vi "General Config.vi"(8 "error In":errorcluster, 9 "DO":T1, 10 "IOList":T3, 11 "reference":refnum<vi>) -> (0 "error out":errorcluster, 3 "Out reference":refnum<vi>)   [LabVIEW 2015]
uses:
  Control Button/Exit.ctl
  Control Button/Daq.ctl
  Control Button/Scanner config.ctl
  Control Button/Program Seq.ctl
  Control Button/Control 1.ctl
  Control Button/cali.ctl
  Control Button/shift change.ctl
  Control Button/User mgt.ctl
  Control Button/model create.ctl
  Data Acquisition/PCI-USB-DAQ/Digital out put.ctl
  Galobal variable_TI.vi
panel:
  out "User Name 3":string
  in  "Model Create":T2
  in  "User Mgt":T4
  out "User Name 2":string
  in  "Shift":T5
  in  "Calibration":T6
  in  "IO List Update":T7
  out "error out 2":errorcluster
  in  "error in (no error)":errorcluster
  in  "Program Seq":T8
  in  "Scanner config":T9
  in  "DAQ Config":T10
  out "User Name":string
  in  "Exit":T11
  out "String":string
  out "appended path":path
  in  "Ring":u16(ring)
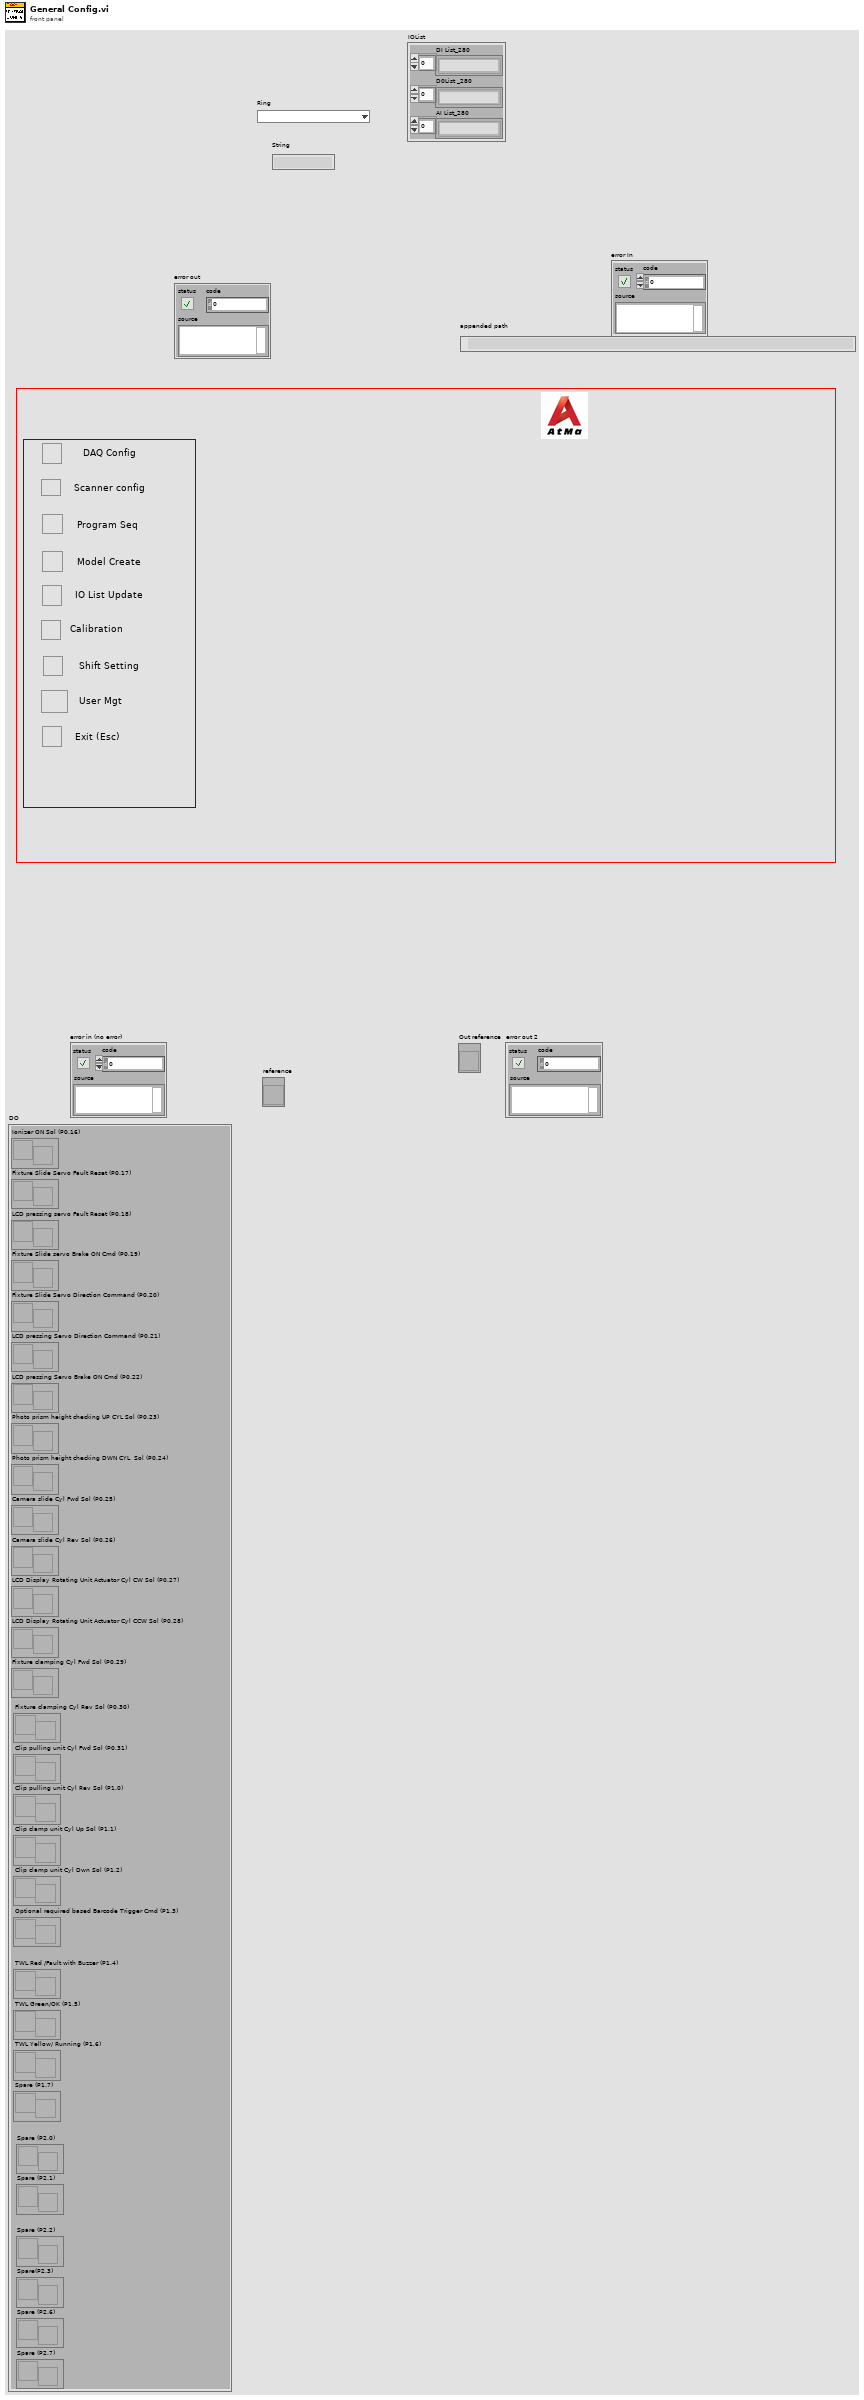
[diagram p1: front panel]
types:
  T1 = typedef "Digital out put.ctl" = cluster{"Ionizer ON Sol (P0.16)":refnum<notifier>, "Fixture Slide Servo Fault Reset (P0.17)":refnum<notifier>, "LCD pressing servo Fault Reset (P0.18)":refnum<notifier>, "Fixture Slide servo Brake ON Cmd (P0.19)":refnum<notifier>, "Fixture Slide Servo Direction Command (P0.20)":refnum<notifier>, "LCD pressing Servo Direction Command (P0.21)":refnum<notifier>, "LCD pressing Servo Brake ON Cmd (P0.22)":refnum<notifier>, "Photo prism height checking UP CYL Sol (P0.23)":refnum<notifier>, "Photo prism height checking DWN CYL  Sol (P0.24)":refnum<notifier>, "Camera slide Cyl Fwd Sol (P0.25)":refnum<notifier>, "Camera slide Cyl Rev Sol (P0.26)":refnum<notifier>, "LCD Display Rotating Unit Actuator Cyl CW Sol (P0.27)":refnum<notifier>, "LCD Display Rotating Unit Actuator Cyl CCW Sol (P0.28)":refnum<notifier>, "Fixture clamping Cyl Fwd Sol (P0.29)":refnum<notifier>, "Fixture clamping Cyl Rev Sol (P0.30)":refnum<notifier>, "Clip pulling unit Cyl Fwd Sol (P0.31)":refnum<notifier>, "Clip pulling unit Cyl Rev Sol (P1.0)":refnum<notifier>, "Clip clamp unit Cyl Up Sol (P1.1)":refnum<notifier>, "Clip clamp unit Cyl Dwn Sol (P1.2)":refnum<notifier>, "Optional required based Barcode Trigger Cmd (P1.3)":refnum<notifier>, "TWL Red /Fault with Buzzer (P1.4)":refnum<notifier>, "TWL Green/OK (P1.5)":refnum<notifier>, "TWL Yellow/ Running (P1.6)":refnum<notifier>, "Spare (P1.7)":refnum<notifier>, "Spare (P2.0)":refnum<notifier>, "Spare (P2.1)":refnum<notifier>, "Spare (P2.2)":refnum<notifier>, "Spare(P2.3)":refnum<notifier>, "Spare (P2.6)":refnum<notifier>, "Spare (P2.7) ":refnum<notifier>}
  T2 = typedef "model create.ctl" = bool
  T3 = cluster{"DI List_280":string[], "D0List _280":string[], "AI List_280":string[]}
  T4 = typedef "User mgt.ctl" = bool
  T5 = typedef "shift change.ctl" = bool
  T6 = typedef "cali.ctl" = bool
  T7 = typedef "Control 1.ctl" = bool
  T8 = typedef "Program Seq.ctl" = bool
  T9 = typedef "Scanner config.ctl" = bool
  T10 = typedef "Daq.ctl" = bool
  T11 = typedef "Exit.ctl" = bool
  T12 = enum32{"Invalid", "Standard", "Closed", "Hidden", "Minimized", "Maximized"}
  T13 = cluster{"XInput":dbl[], "Y New Value":dbl[], "Avg point":i16}[]
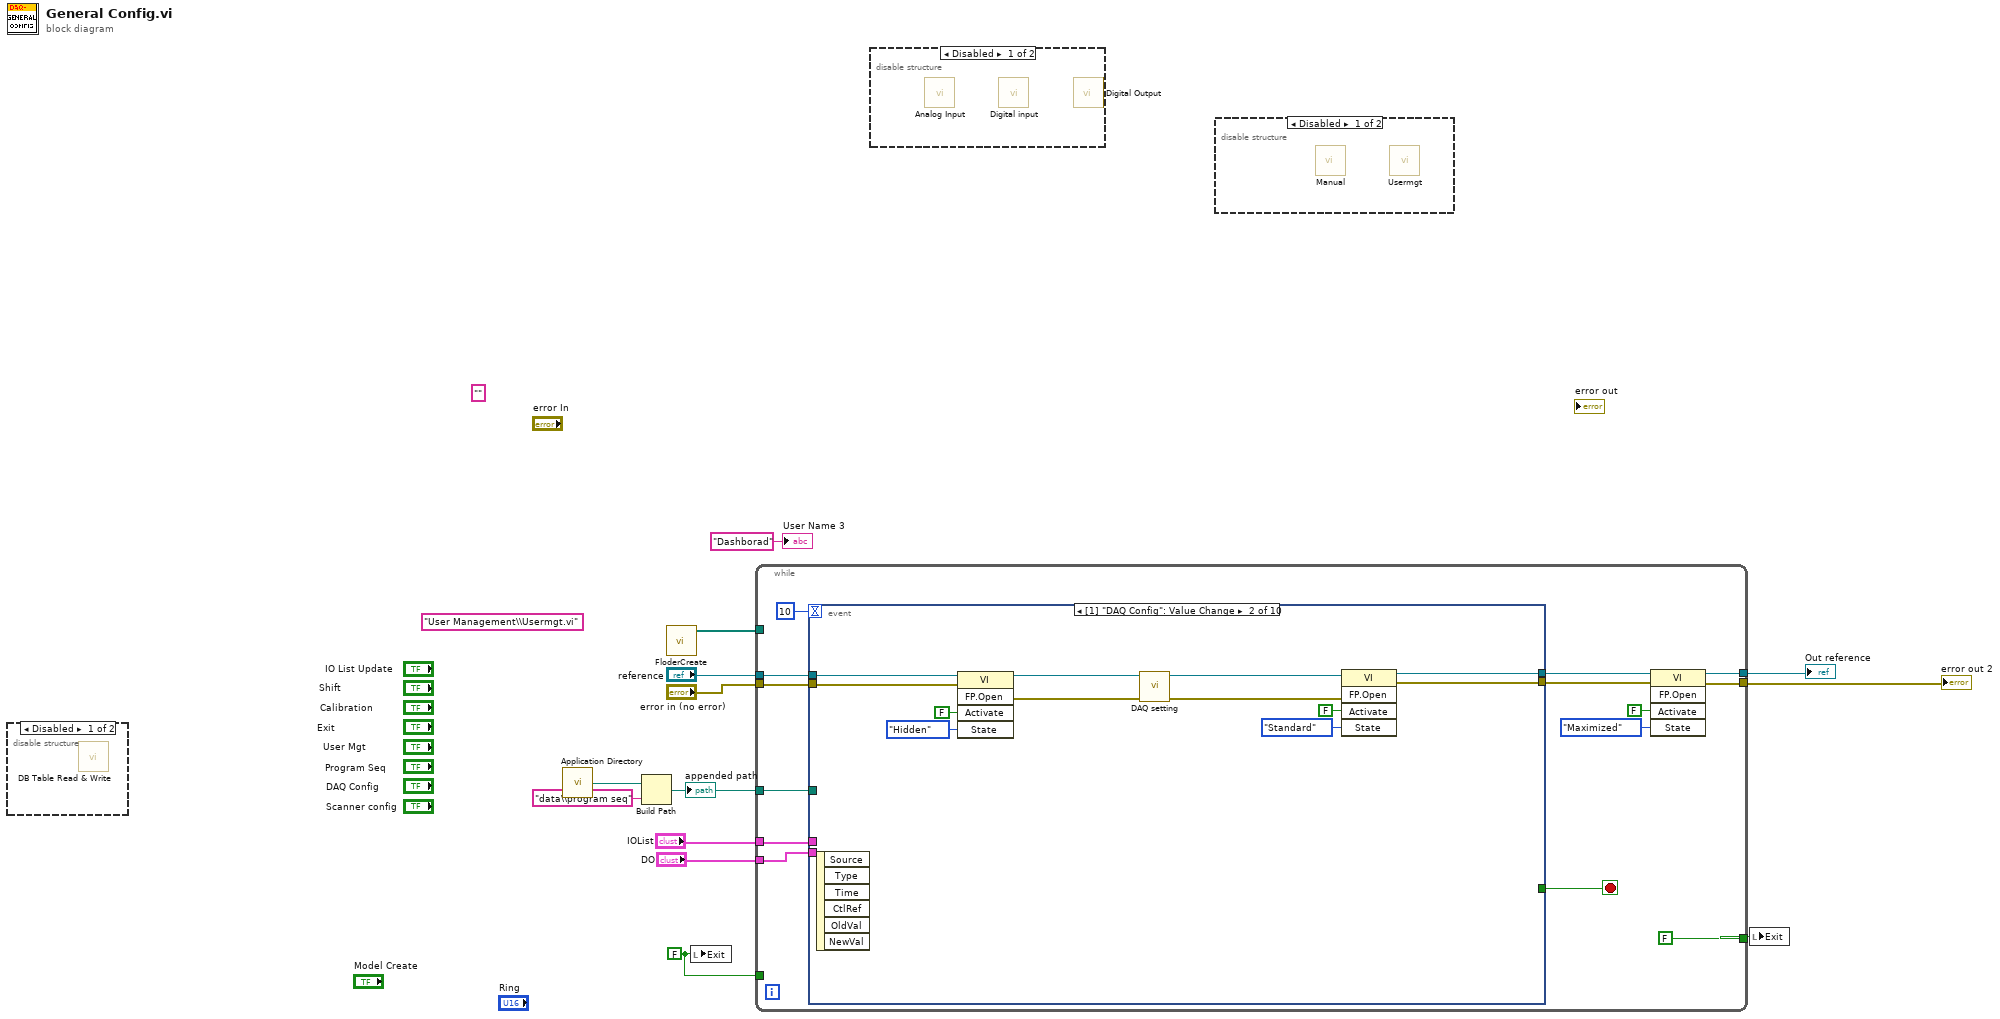
[diagram p0: block diagram]
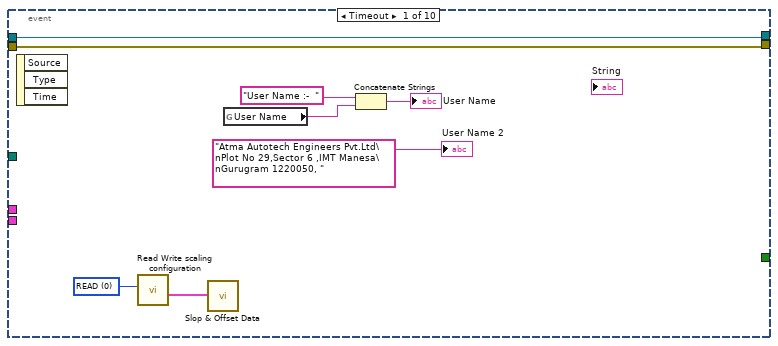
[diagram p5: hidden frame]
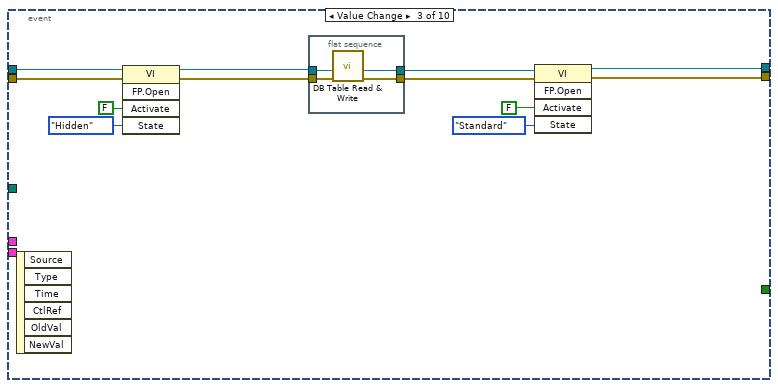
[diagram p6: hidden frame]
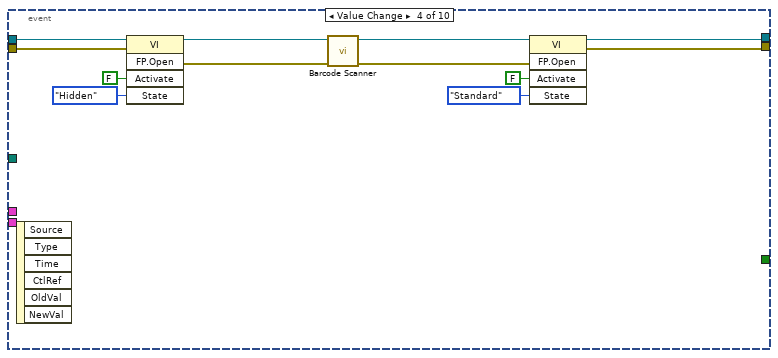
[diagram p7: hidden frame]
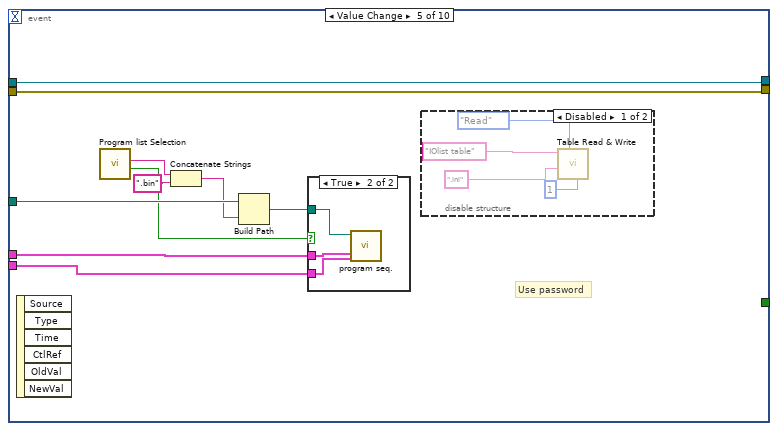
[diagram p8: hidden frame]
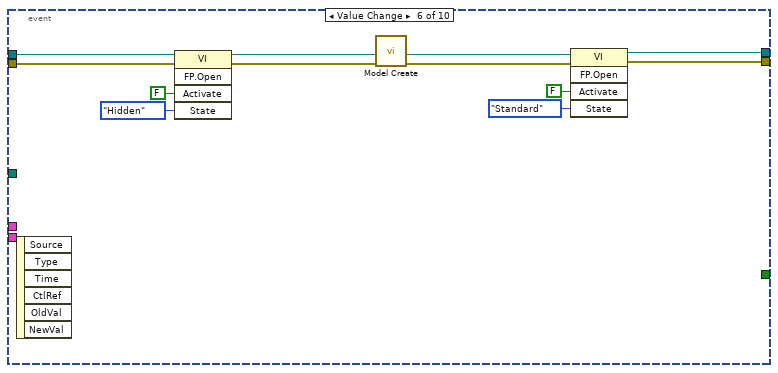
[diagram p11: hidden frame]
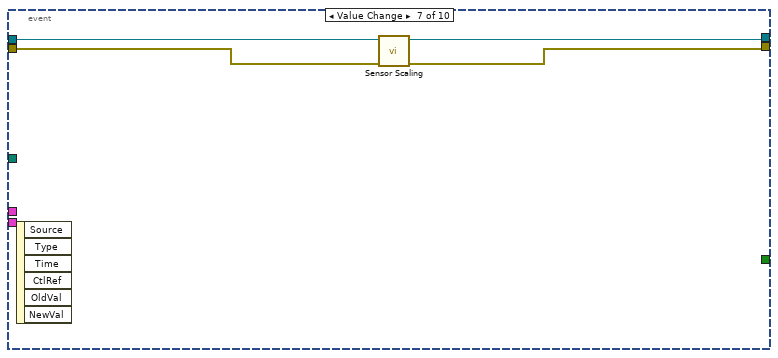
[diagram p12: hidden frame]
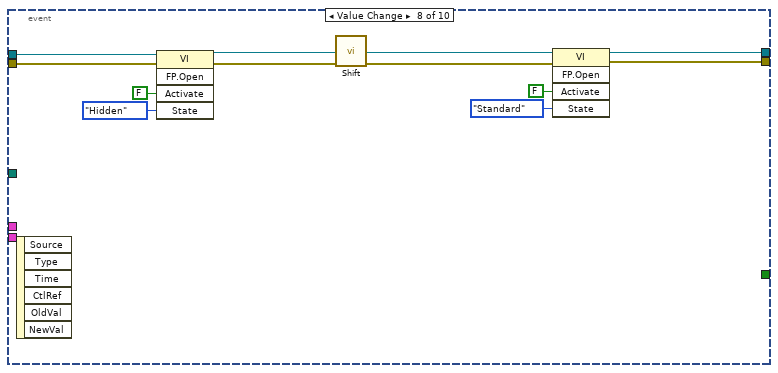
[diagram p13: hidden frame]
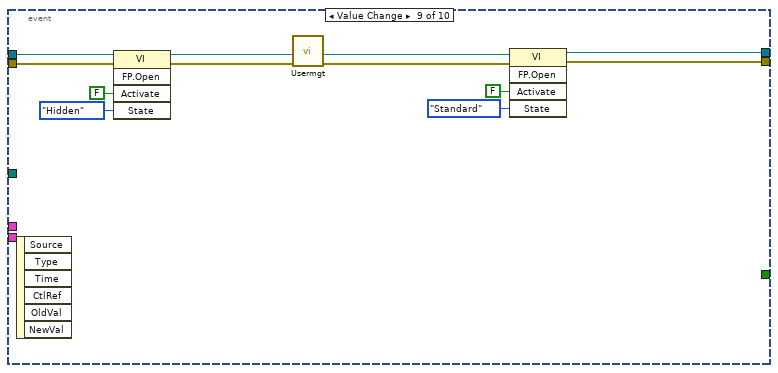
[diagram p14: hidden frame]
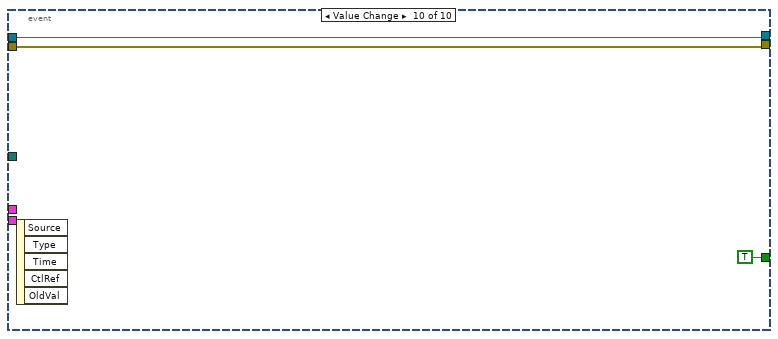
[diagram p15: hidden frame]
diagram:
  w10 = T11 FALSE ("Exit")
  (unwired) "User Management\\Usermgt.vi" ("name or relative path")
  (unwired) ""
  n1 = disable-structure shown="Disabled" {
    frame Disabled {
      n2 = call "DB Table Read & Write.vi"() -> ()  [unwired: 10 in, 2 out]
    }
    frame Enabled {
    }
  }
  n3 = call <vilib>:"Application Directory.vi"() -> ("Application Directory"=w6:path)
  n4 = Build Path(base path=w6, name or relative path="data\\program seq") -> (appended path=w3:path)
  "appended path" <- w3
  n5 = call "FloderCreate.vi"() -> ("File Path"=w7:path[])  [unwired: 11 in]
  n6 = local write "Exit"(w10) -> ()
  n7 = while {
    tunnel: w3 -> [w15]
    tunnel: "reference" -> [w25]
    tunnel: "error in (no error)" -> [w24]
    tunnel: [w19] -> w12
    tunnel: [w18] -> w11
    tunnel: w10 -> [_]
    tunnel: [T11 FALSE ("Exit")] -> w9
    tunnel: w7 -> [_]
    tunnel: "IOList" -> [w16]
    tunnel: "DO" -> [w14]
    stop <- w26 stop-if-true
    n8 = event shown="[1] \"DAQ Config\": Value Change" {
      selector: _ -> [_ _ _ _ _ _ _ _ _ _]
      dyn-events: _ -> [_ _ _ _ _ _ _ _ _ _]
      timeout: 10 -> [_ _ _ _ _ _ _ _ _ _]
      tunnel: [_ _ _ _ _ _ _ _ _ TRUE ("Exit")] -> w26
      tunnel: w25 -> [w32 w39 w51 w73 w85 w99 w106 w114 w123 w131]
      tunnel: w24 -> [w31 w38 w50 w72 w84 w98 w105 w112 w121 w130]
      tunnel: [w32 w37 w58 w65 w85 w94 w106 w113 w122 w131] -> w21
      tunnel: [w31 w36 w57 w64 w84 w93 w104 w111 w120 w130] -> w20
      tunnel: w16 -> [_ _ _ _ w83 _ _ _ _ _]
      tunnel: w15 -> [_ _ _ _ w82 _ _ _ _ _]
      tunnel: w14 -> [_ _ _ _ w76 _ _ _ _ _]
      event Timeout {
        w30 = u16 0 items=["READ", "WRITE"] ("Read/Write")
        n9 = event-data() -> ()  [unwired: 1 in, 3 out]
        n10 = call "Read Write scaling configuration.vi"("Read/Write"=w30) -> ("Output"=w29:T13)  [unwired: 4 in, 2 out]
        n11 = call "Slop & Offset Data.vi"("Input"=w29) -> ()  [unwired: 10 in, 1 out]
        n12 = global read "Galobal variable_TI.vi" "User Name"() -> (w35:string)
        n13 = Concatenate Strings("User Name :-  " ("string"), w35) -> (→"User Name":string)
        "User Name 2" <- "Atma Autotech Engineers Pvt.Ltd\nPlot No 29,Sector 6 ,IMT Manesa\nGurugram 1220050, " ("string")
      }
      event Value Change {
        n14 = event-data() -> ()  [unwired: 1 in, 6 out]
        n15 = invoke class="VI" method="FP.Open"(reference=w39, error in=w38, "Activate"=FALSE ("Activate?"), "State"=T12."Hidden") -> (reference out=w45:refnum<vi>, error out=w44:errorcluster)  [unwired: 1 in, 3 out]
        n16 = call "DAQ setting.vi"("error in (no error)"=w44, "vi reference"=w45) -> ("error Out"=w40:errorcluster, "Out reference"=w41:refnum<vi>)  [unwired: 8 in]
        n17 = invoke class="VI" method="FP.Open"(reference=w41, error in=w40, "Activate"=FALSE ("Activate?"), "State"=T12."Standard") -> (reference out=w37:refnum<vi>, error out=w36:errorcluster)  [unwired: 1 in, 3 out]
      }
      event Value Change {
        n18 = event-data() -> ()  [unwired: 1 in, 6 out]
        n19 = invoke class="VI" method="FP.Open"(reference=w51, error in=w50, "Activate"=FALSE ("Activate?"), "State"=T12."Hidden") -> (reference out=w49:refnum<vi>, error out=w48:errorcluster)  [unwired: 1 in, 3 out]
        n20 = flat-sequence {
          tunnel: [w60] -> w55
          tunnel: [w61] -> w54
          tunnel: w49 -> [w62]
          tunnel: w48 -> [w63]
          frame #0 {
            n21 = call "DB Table Read & Write.vi"("error in"=w63, "reference"=w62) -> ("error out"=w60:errorcluster, "referenceOut"=w61:refnum<vi>)  [unwired: 8 in]
          }
        }
        n22 = invoke class="VI" method="FP.Open"(reference=w54, error in=w55, "Activate"=FALSE ("Activate?"), "State"=T12."Standard") -> (reference out=w58:refnum<vi>, error out=w57:errorcluster)  [unwired: 1 in, 3 out]
      }
      event Value Change {
        n23 = event-data() -> ()  [unwired: 1 in, 6 out]
        n24 = invoke class="VI" method="FP.Open"(reference=w73, error in=w72, "Activate"=FALSE ("Activate?"), "State"=T12."Hidden") -> (reference out=w69:refnum<vi>, error out=w68:errorcluster)  [unwired: 1 in, 3 out]
        n25 = call "Barcode Scanner.vi"("error in (no error)"=w68, "reference"=w69) -> ("error in (no error) 2"=w66:errorcluster, "reference 2"=w67:refnum<vi>)  [unwired: 8 in]
        n26 = invoke class="VI" method="FP.Open"(reference=w67, error in=w66, "Activate"=FALSE ("Activate?"), "State"=T12."Standard") -> (reference out=w65:refnum<vi>, error out=w64:errorcluster)  [unwired: 1 in, 3 out]
      }
      event Value Change {
        # "Use password"
        n27 = event-data() -> ()  [unwired: 1 in, 6 out]
        n28 = call "Program list Selection.vi"() -> ("Exit"=w77:bool, "String"=w78:string)  [unwired: 10 in]
        n29 = Concatenate Strings(w78, ".bin" ("string")) -> (w81:string)
        n30 = Build Path(base path=w82, name or relative path=w81) -> (appended path=w79:path)
        n31 = case shown="True" w77 {
          tunnel: w83 -> [_ w86]
          tunnel: w79 -> [_ w88]
          tunnel: w76 -> [_ w87]
          frame False {
          }
          frame True {
            n32 = call "program seq..vi"("IOList"=w86, "DO"=w87, "Filepath"=w88) -> ()  [unwired: 8 in, 1 out]
          }
        }
        n33 = disable-structure shown="Disabled" {
          frame Disabled {
            n34 = call "Table Read & Write.vi"("File Name"="IOlist table", "File type"=".ini", "Enum"=enum16{"Read", "Write"}."Read", "index"=1) -> ()  [unwired: 5 in, 2 out]
          }
          frame Enabled {
          }
        }
      }
      event Value Change {
        n35 = event-data() -> ()  [unwired: 1 in, 6 out]
        n36 = invoke class="VI" method="FP.Open"(reference=w99, error in=w98, "Activate"=FALSE ("Activate?"), "State"=T12."Hidden") -> (reference out=w95:refnum<vi>, error out=w97:errorcluster)  [unwired: 1 in, 3 out]
        n37 = call "Model Create.vi"("error in (no error)"=w97) -> ("error out"=w96:errorcluster)  [unwired: 10 in]
        n38 = invoke class="VI" method="FP.Open"(reference=w95, error in=w96, "Activate"=FALSE ("Activate?"), "State"=T12."Standard") -> (reference out=w94:refnum<vi>, error out=w93:errorcluster)  [unwired: 1 in, 3 out]
      }
      event Value Change {
        n39 = event-data() -> ()  [unwired: 1 in, 6 out]
        n40 = call "Sensor Scaling.vi"("error in"=w105) -> ("error out"=w104:errorcluster)  [unwired: 9 in, 1 out]
      }
      event Value Change {
        n41 = event-data() -> ()  [unwired: 1 in, 6 out]
        n42 = invoke class="VI" method="FP.Open"(reference=w114, error in=w112, "Activate"=FALSE ("Activate?"), "State"=T12."Hidden") -> (reference out=w115:refnum<vi>, error out=w117:errorcluster)  [unwired: 1 in, 3 out]
        n43 = call "Shift.vi"("error in"=w117) -> ("error out"=w116:errorcluster)  [unwired: 10 in]
        n44 = invoke class="VI" method="FP.Open"(reference=w115, error in=w116, "Activate"=FALSE ("Activate?"), "State"=T12."Standard") -> (reference out=w113:refnum<vi>, error out=w111:errorcluster)  [unwired: 1 in, 3 out]
      }
      event Value Change {
        n45 = event-data() -> ()  [unwired: 1 in, 6 out]
        n46 = invoke class="VI" method="FP.Open"(reference=w123, error in=w121, "Activate"=FALSE ("Activate?"), "State"=T12."Hidden") -> (reference out=w124:refnum<vi>, error out=w119:errorcluster)  [unwired: 1 in, 3 out]
        n47 = call "Usermgt.vi"("error In"=w119) -> ("error out"=w118:errorcluster)  [unwired: 10 in]
        n48 = invoke class="VI" method="FP.Open"(reference=w124, error in=w118, "Activate"=FALSE ("Activate?"), "State"=T12."Standard") -> (reference out=w122:refnum<vi>, error out=w120:errorcluster)  [unwired: 1 in, 3 out]
      }
      event Value Change {
        n49 = event-data() -> ()  [unwired: 1 in, 5 out]
      }
    }
    n50 = invoke class="VI" method="FP.Open"(reference=w21, error in=w20, "Activate"=FALSE ("Activate?"), "State"=T12."Maximized") -> (reference out=w19:refnum<vi>, error out=w18:errorcluster)  [unwired: 1 in, 3 out]
  }
  "Out reference" <- w12
  "error out 2" <- w11
  n51 = disable-structure shown="Disabled" {
    frame Disabled {
      n52 = call "Analog Input.vi"() -> ()  [unwired: 10 in, 2 out]
      n53 = call "Digital input.vi"() -> ()  [unwired: 10 in, 2 out]
      n54 = call "Digital Output.vi"() -> ()  [unwired: 10 in, 2 out]
    }
    frame Enabled {
    }
  }
  n55 = disable-structure shown="Disabled" {
    frame Disabled {
      n56 = call "Manual.vi"() -> ()  [unwired: 10 in, 2 out]
      n57 = call "Usermgt.vi"() -> ()  [unwired: 11 in, 1 out]
    }
    frame Enabled {
    }
  }
  n58 = local write "Exit"(w9) -> ()
  "User Name 3" <- "Dashborad" ("User Name 3")
